vi "File_Build Path from File Data.vi"(11 "File Data":T1) -> (3 "appended path":path)   [LabVIEW 2021]
uses:
  TypeDefs/Cluster_IconFilename.ctl
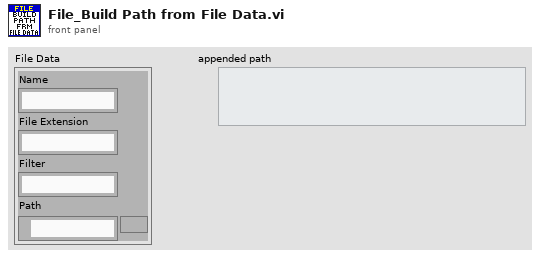
[diagram p1: front panel]
types:
  T1 = typedef "Cluster_IconFilename.ctl" = cluster{"Name":string, "File Extension  ":string, "Filter":string, "Path":path}
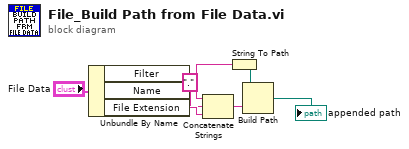
[diagram p0: block diagram]
diagram:
  n1 = Unbundle By Name("File Data") -> ("Filter"=w6:string, "Name"=w7:string, "File Extension"=w8:string)
  n2 = Concatenate Strings(w7, "." ("string"), w8) -> (w1:string)
  n3 = String To Path(string=w6) -> (path=w3:path)
  n4 = Build Path(base path=w3, name or relative path=w1) -> (appended path=→"appended path":path)
